vi "Get SPI Channel Name.vi"(7 "SPI Channel Names":string[](array[string])=["A/SPI", "B/SPI"], 8 "Error In":errorcluster, 10 "SPI Channel":u8) -> (0 "Error Out":errorcluster, 2 "myRIO SPI Channel":string="A/SPI")   [LabVIEW 2011, in "LVH-LINX.lvlib" / "myRIO.lvlib"]
doc: "Get myRIO SPI Channel Names From Channel Number"
uses:
  myRIO.lvlib
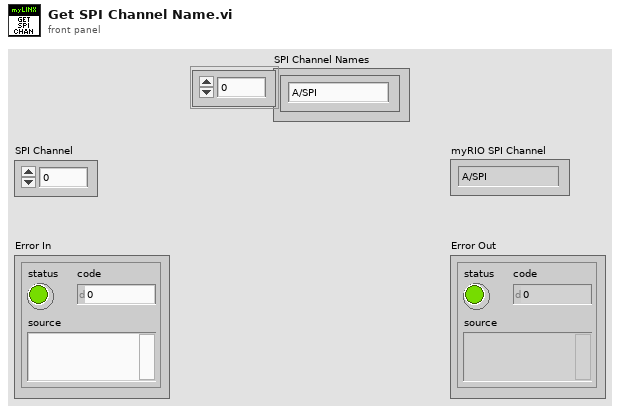
[diagram p1: front panel]
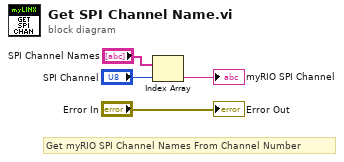
[diagram p0: block diagram]
diagram:
  # "Get myRIO SPI Channel Names From Channel Number"
  n1 = Index Array(array="SPI Channel Names", index="SPI Channel") -> (element=→"myRIO SPI Channel":string)
  "Error Out" <- "Error In"
